vi "Add Timestamp to DB.vi"(8 "error in (no error)":errorcluster, 10 "Timestamp":T1, 11 "TimeStamper in":refnum<class "TimeStamper.lvclass">) -> (0 "error out":errorcluster, 3 "TimeStamper out":refnum<class "TimeStamper.lvclass">)   [LabVIEW 2014, in "TimeStamper.lvclass"]
uses:
  TimeStamper.lvclass
  AcquistionObject/AcquistionObject.lvclass
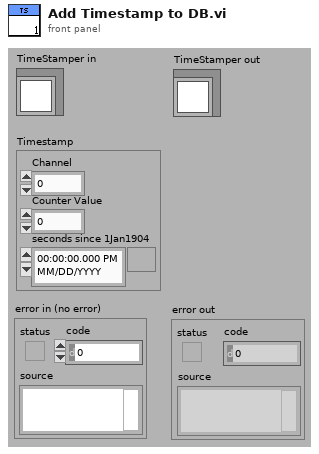
[diagram p1: front panel]
types:
  T1 = cluster{"Channel":i32, "Counter Value":u32, "seconds since 1Jan1904":timestamp}
  T2 = cluster{"setup":u8, "subject_id":u64, "session_start_time":dbl, "channel":u64, "counter":u64, "time":u64}
  T3 = typedef "NI_Database_API.lvlib/Conn ObjectReference.ctl" = refnum<k1>
  T4 = typedef "SessionPrimary.ctl" = cluster{"setup":u8, "subject_id":i32, "session_start_time":dbl}
  T5 = cluster{"reference":T3, "table":string, "columns":string[], i32}
  T6 = cluster{cluster{"reference":T3, "table":string, "columns":string[], i32}, "Variant":variant}
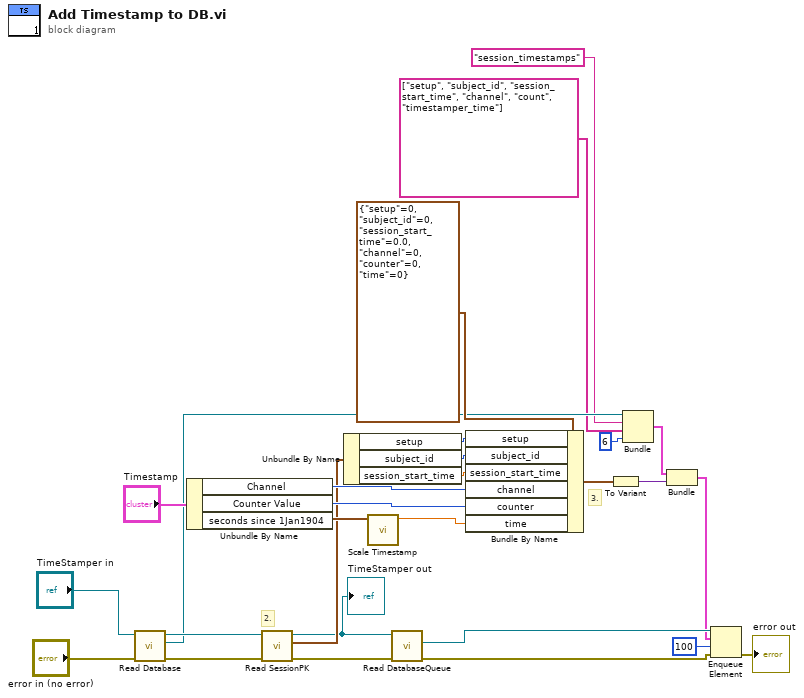
[diagram p0: block diagram]
diagram:
  # "2."
  # "3."
  n1 = call-dynamic "Read Database.vi"("error in (no error)"="error in (no error)", "AcquistionObject in"="TimeStamper in") -> ("error out"=w17:errorcluster, "reference"=w14:T3, "AcquistionObject out"=w15:refnum<class "TimeStamper.lvclass">)  [unwired: 7 in]
  n2 = Unbundle By Name("Timestamp") -> ("Channel"=w22:i32, "Counter Value"=w21:u32, "seconds since 1Jan1904"=w20:timestamp)
  n3 = call-dynamic "Read SessionPK.vi"("error in (no error)"=w17, "TimeStamper in"=w15) -> ("error out"=w11:errorcluster, "SessionPK"=w16:T4, "TimeStamper out"=w6:refnum<class "TimeStamper.lvclass">)  [unwired: 7 in]
  "TimeStamper out" <- w6
  n4 = Unbundle By Name(w16) -> ("setup"=w28:u8, "subject_id"=w27:i32, "session_start_time"=w18:dbl)
  n5 = call "Scale Timestamp.vi"("Time Stamp"=w20) -> ("Scaled timestamp"=w19:dbl)  [unwired: 10 in]
  n6 = call-dynamic "Read DatabaseQueue.vi"("error in (no error)"=w11, "AcquistionObject in"=w6) -> ("error out"=w10:errorcluster, "DatabaseQueue"=w8:refnum<queue>)  [unwired: 7 in, 1 out]
  n7 = Bundle By Name(cluster=T2 {"setup"=0, "subject_id"=0, "session_start_time"=0.0, "channel"=0, "counter"=0, "time"=0} ("Cluster"), "setup"=w28, "subject_id"=w27, "session_start_time"=w18, "channel"=w22, "counter"=w21, "time"=w19) -> (w4:T2)
  n8 = To Variant(anything=w4) -> (Variant=w2:variant)
  n9 = Bundle("reference"=w14, "table"="session_timestamps", "columns"=string[] ["setup", "subject_id", "session_start_time", "channel", "count", "timestamper_time"], 6) -> (w3:T5)  [unwired: 1 in]
  n10 = Bundle(w3, "Variant"=w2) -> (w1:T6)  [unwired: 1 in]
  n11 = Enqueue Element(queue=w8, element=w1, timeout in ms (-1)=100, error in (no error)=w10) -> (error out=→"error out":errorcluster)  [unwired: 2 out]
